vi "F Dwf Digital Out Data Set.vi"(7 "countOfBits":u32, 8 "error in (no error)":errorcluster, 9 "rgBits":u8[](array[numeric]), 10 "idxChannel":i32, 11 "hdwf":i32) -> (0 "error out":errorcluster, 3 "function return":i32)   [LabVIEW 2021, in "Olasdwf.lvlib"]
doc: "DWFAPI int FDwfDigitalOutDataSet(HDWF hdwf, int idxChannel, void *rgBits, unsigned int countOfBits);"
uses:
  Olasdwf.lvlib
  Windows/System32/dwf.dll
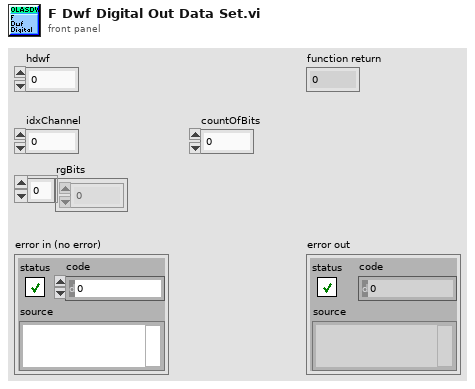
[diagram p1: front panel]
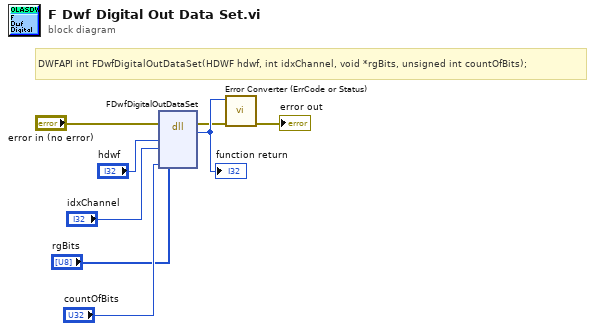
[diagram p0: block diagram]
diagram:
  # "DWFAPI int FDwfDigitalOutDataSet(HDWF hdwf, int idxChannel, void *rgBits, unsigned int countOfBits);"
  n1 = dll-call lib="/Windows/System32/dwf.*" fn="FDwfDigitalOutDataSet"(error in="error in (no error)", "hdwf"="hdwf", "idxChannel"="idxChannel", "rgBits"="rgBits", "countOfBits"="countOfBits") -> (error out=w3:errorcluster, "return type"=w8:i32)  [unwired: 6 in, 1 out]
  "function return" <- w8
  n2 = call "Error Converter (ErrCode or Status).vi"("error in (no error)"=w3, "error code"=w8) -> ("error out"=→"error out":errorcluster)  [unwired: 9 in]
